vi "CreateBeamLineNode.vi"(8 "Error In":errorcluster, 10 "Experiment":T1={"File Path"=path "", "Operator"="Operator", "Project"="Project Description", "Target Dose (dpa)"=0.0, "Sample"={"Name"="", "Description"="", "Molar Mass (g/mol)"=0.0, "Density (g/cm^3)"=0.0, "Irradiation Area (cm^2)"=0.0, "SRIM Damage Peak (disp * ions/cm)"=0.0}, "Beam Line"={"Type"=enum."Ion Beam Analysis", "Ion"=enum."H", "Charge State"=0, "Total Source Ion Energy (kV)"=nan}, "Runs"=[]} {"Beam Line"."Charge State" min=1}, 11 "DOM Document In":refnum<k20>) -> (0 "Error out":errorcluster, 2 "Beam Line Node":refnum<k20>, 3 "DOM Document Out":refnum<k20>)   [LabVIEW 2012]
uses:
  Experiment.ctl
  Sample.ctl
  BeamLine.ctl
  BeamLineType.ctl
  BeamLineIon.ctl
  ExperimentRun.ctl
  ExperimentRunTiming.ctl
  ExperimentRunDose.ctl
  ExperimentRunFluence.ctl
  ExperimentRunTotalCharge.ctl
  <resource>/objmgr/DOMUserDefRef.rc
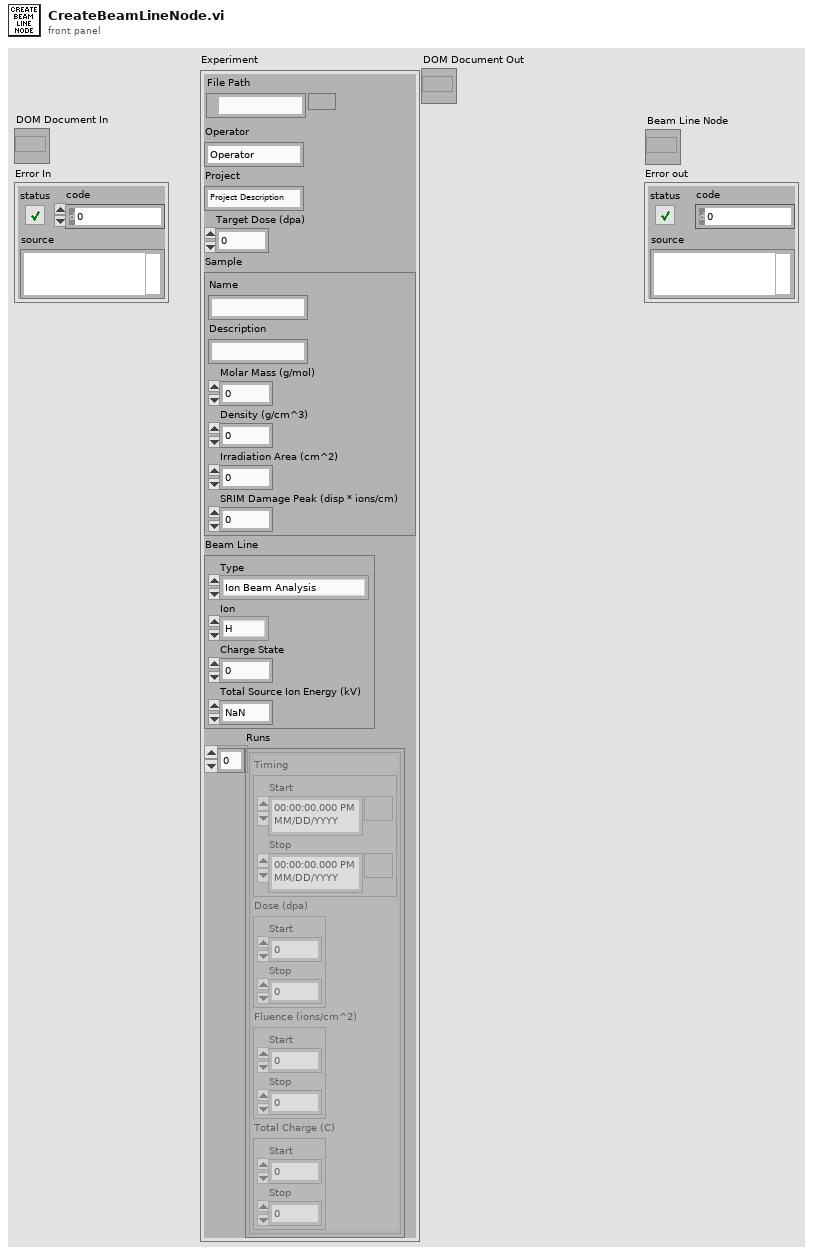
[diagram p1: front panel]
types:
  T1 = typedef "Experiment.ctl" = cluster{"File Path":path, "Operator":string, "Project":string, "Target Dose (dpa)":dbl, "Sample":T2, "Beam Line":T3, "Runs":T6[]}
  T2 = typedef "Sample.ctl" = cluster{"Name":string, "Description":string, "Molar Mass (g/mol)":dbl, "Density (g/cm^3)":dbl, "Irradiation Area (cm^2)":dbl, "SRIM Damage Peak (disp * ions/cm)":dbl}
  T3 = typedef "BeamLine.ctl" = cluster{"Type":T4, "Ion":T5, "Charge State":u8, "Total Source Ion Energy (kV)":dbl}
  T4 = typedef "BeamLineType.ctl" = enum16{"Ion Beam Analysis", "Auxiliary", "Radiation Damage"}
  T5 = typedef "BeamLineIon.ctl" = enum16{"H", "He", "C", "Fe", "Ni", "Pt", "Si", "Ag", "Au"}
  T6 = typedef "ExperimentRun.ctl" = cluster{"Timing":T7, "Dose (dpa)":T8, "Fluence (ions/cm^2)":T9, "Total Charge (C)":T10}
  T7 = typedef "ExperimentRunTiming.ctl" = cluster{"Start":timestamp, "Stop":timestamp}
  T8 = typedef "ExperimentRunDose.ctl" = cluster{"Start":dbl, "Stop":dbl}
  T9 = typedef "ExperimentRunFluence.ctl" = cluster{"Start":dbl, "Stop":dbl}
  T10 = typedef "ExperimentRunTotalCharge.ctl" = cluster{"Start":dbl, "Stop":dbl}
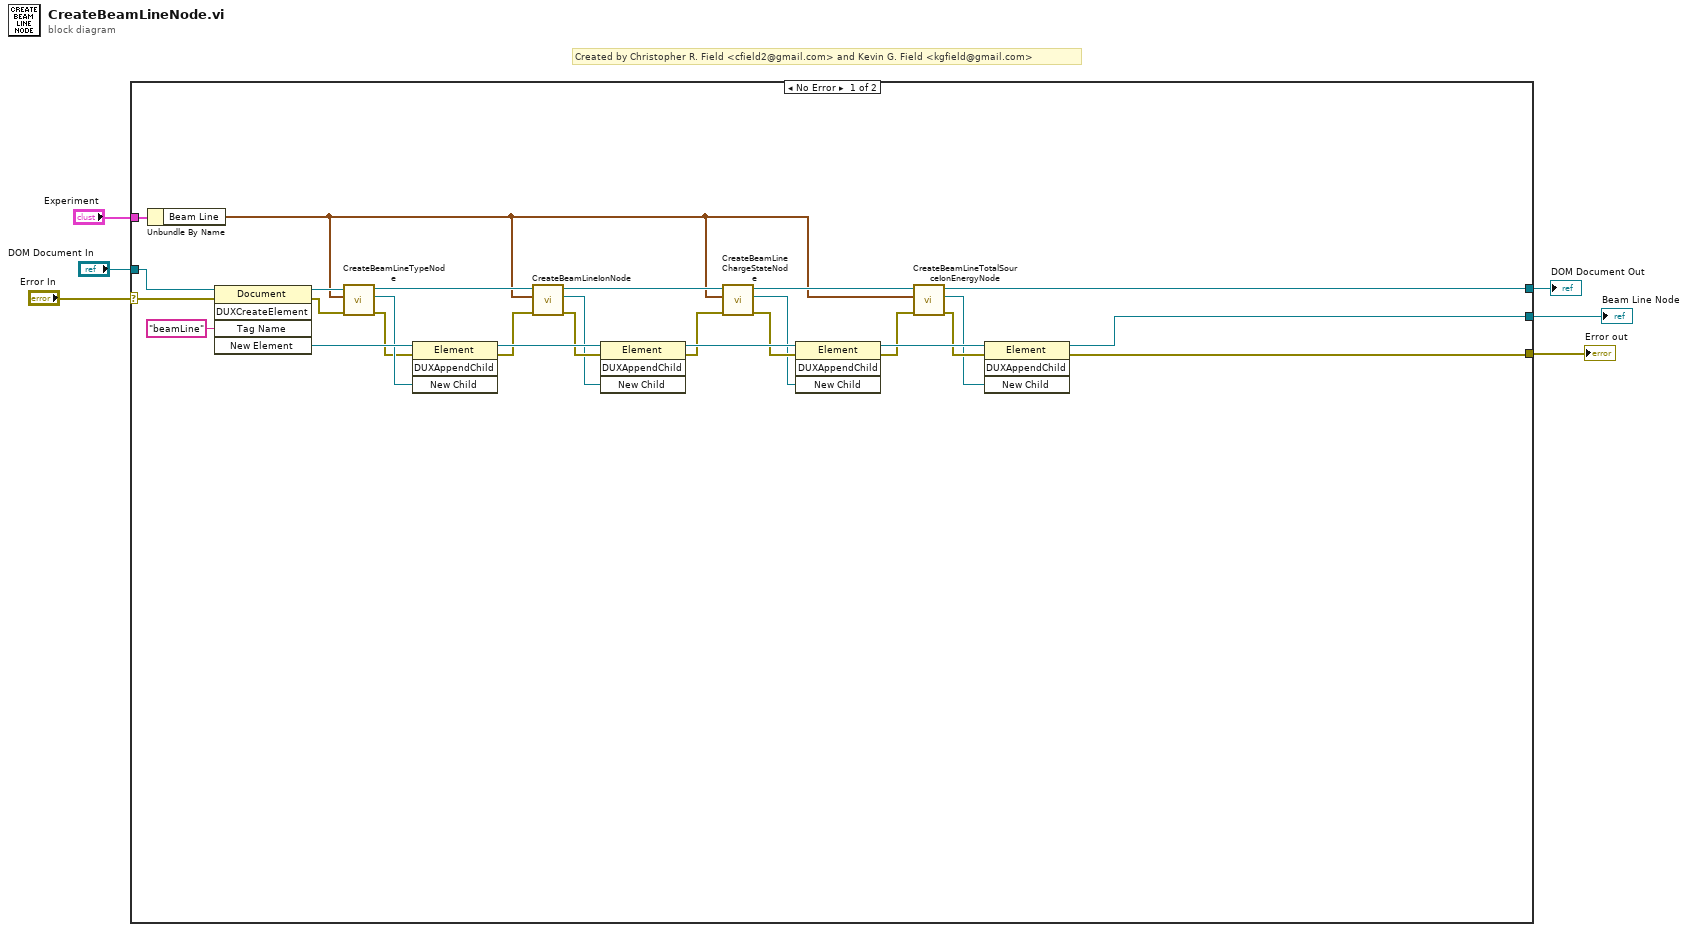
[diagram p0: block diagram]
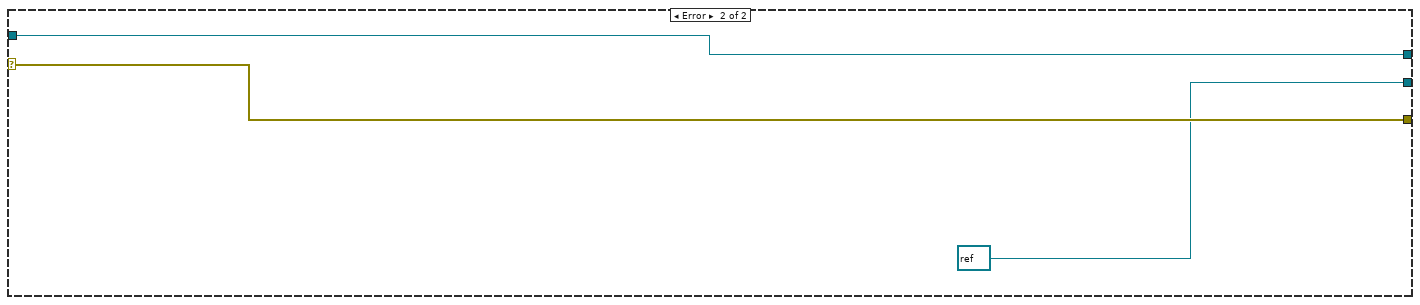
[diagram p2: hidden frame]
diagram:
  # "Created by Christopher R. Field <cfield2@gmail.com> and Kevin G. Field <kgfield@gmail.com>"
  n1 = case shown="No Error" "Error In" {
    selector: "Error In" -> [w31 w36]
    tunnel: "DOM Document In" -> [w34 w37]
    tunnel: [w8 refnum<k20> refnum ("Operator Node 2")] -> w5
    tunnel: [w7 w36] -> w4
    tunnel: "Experiment" -> [w32 _]
    tunnel: [w9 w37] -> w1
    frame No Error {
      n2 = Unbundle By Name(w32) -> ("Beam Line"=w13:T3)
      n3 = invoke class="Document" method="DUXCreateElement"(reference=w34, error in=w31, "Tag Name"="beamLine") -> (reference out=w26:refnum<k20>, error out=w25:errorcluster, "New Element"=w30:refnum<k20>)  [unwired: 2 in, 2 out]
      n4 = call "CreateBeamLineTypeNode.vi"("Error In"=w25, "Beam Line"=w13, "DOM Document In"=w26) -> ("Error out"=w23:errorcluster, "Beam Line Type Node"=w24:refnum<k20>, "DOM Document Out"=w22:refnum<k20>)  [unwired: 6 in]
      n5 = invoke class="Element" method="DUXAppendChild"(reference=w30, error in=w23, "New Child"=w24) -> (reference out=w29:refnum<k20>, error out=w21:errorcluster)  [unwired: 1 in, 2 out]
      n6 = call "CreateBeamLineIonNode.vi"("Error In"=w21, "Beam Line"=w13, "DOM Document In"=w22) -> ("Error out"=w20:errorcluster, "Beam Line Ion Node"=w19:refnum<k20>, "DOM Document Out"=w18:refnum<k20>)  [unwired: 6 in]
      n7 = invoke class="Element" method="DUXAppendChild"(reference=w29, error in=w20, "New Child"=w19) -> (reference out=w28:refnum<k20>, error out=w17:errorcluster)  [unwired: 1 in, 2 out]
      n8 = call "CreateBeamLineChargeStateNode.vi"("Error In"=w17, "Beam Line"=w13, "DOM Document In"=w18) -> ("Error out"=w16:errorcluster, "Beam Line Charge State Node"=w15:refnum<k20>, "DOM Document Out"=w14:refnum<k20>)  [unwired: 6 in]
      n9 = invoke class="Element" method="DUXAppendChild"(reference=w28, error in=w16, "New Child"=w15) -> (reference out=w27:refnum<k20>, error out=w12:errorcluster)  [unwired: 1 in, 2 out]
      n10 = call "CreateBeamLineTotalSourceIonEnergyNode.vi"("Error In"=w12, "Beam Line"=w13, "DOM Document In"=w14) -> ("Error out"=w11:errorcluster, "Beam Line Total Source Ion Energy Node"=w10:refnum<k20>, "DOM Document Out"=w9:refnum<k20>)  [unwired: 6 in]
      n11 = invoke class="Element" method="DUXAppendChild"(reference=w27, error in=w11, "New Child"=w10) -> (reference out=w8:refnum<k20>, error out=w7:errorcluster)  [unwired: 1 in, 2 out]
    }
    frame Error {
    }
  }
  "Beam Line Node" <- w5
  "Error out" <- w4
  "DOM Document Out" <- w1
